vi "integrator.vi"(11 "y":fxp<+/-,24,24>) -> (3 "Numeric":fxp<+/-,24,24>)   [LabVIEW 2013]
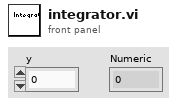
[diagram p1: front panel]
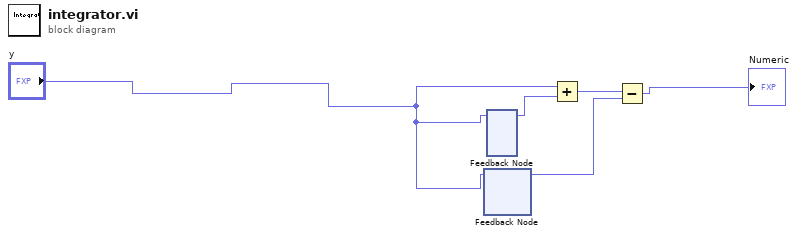
[diagram p0: block diagram]
diagram:
  n1 = feedback #1() -> (w4:fxp<+/-,24,24>)  [unwired: 1 in]
  n2 = feedback-in #1("y") -> ()
  n3 = feedback #2() -> (w1:fxp<+/-,24,24>)  [unwired: 1 in]
  n4 = feedback-in #2("y") -> ()
  n5 = Add(x="y", y=w1) -> (x+y=w3:fxp<+/-,24,24>)
  n6 = Subtract(x=w3, y=w4) -> (x-y=→"Numeric":fxp<+/-,24,24>)
